vi "Delete.vi"(8 "error in":errorcluster, 11 "Driver path":path) -> (0 "error out":errorcluster)   [LabVIEW 2020, in "r307-python-labview-driver.lvlib"]
uses:
  r307-python-labview-driver.lvlib
  <vilib>/Utility/error.llb/whitespace.ctl
panel:
  out "standard error":string
  out "standard output":string
  in  "Enrolled ID":u32
  out "Deleted":bool
  out "command line":string="cmc /c python \"%s\" ENROLL"
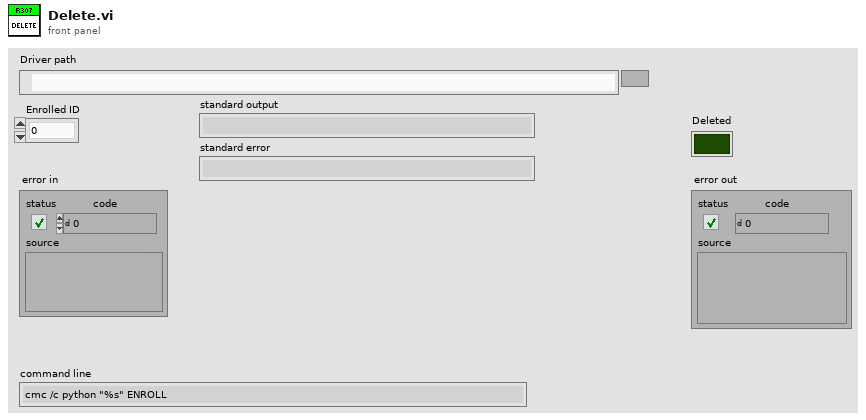
[diagram p1: front panel]
types:
  T1 = typedef "whitespace.ctl" = u16
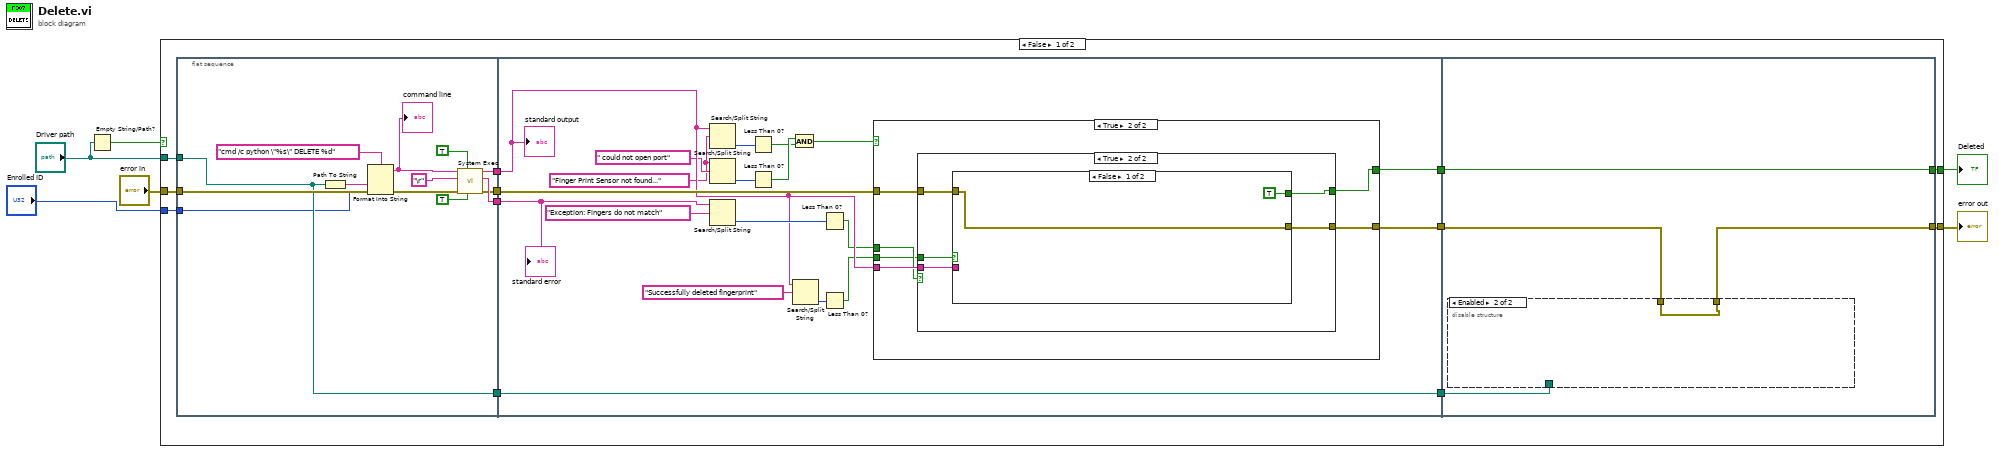
[diagram p0: block diagram]
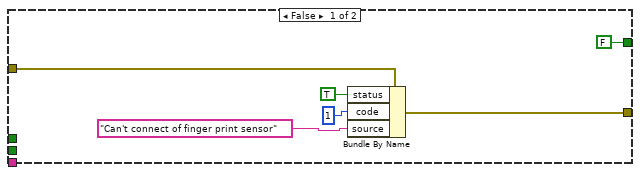
[diagram p2: hidden frame]
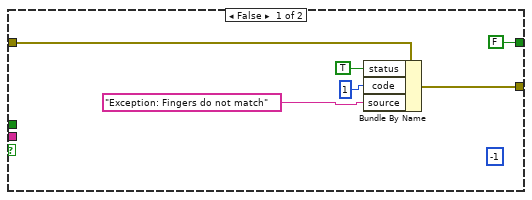
[diagram p3: hidden frame]
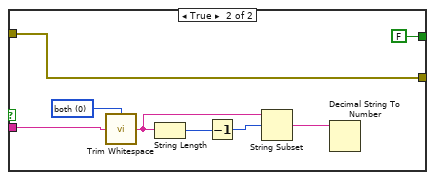
[diagram p4: hidden frame]
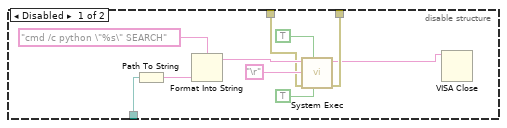
[diagram p5: hidden frame]
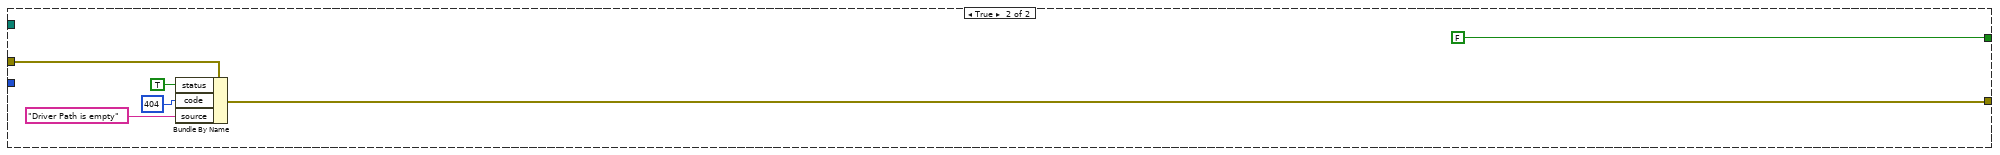
[diagram p6: hidden frame]
diagram:
  n1 = Empty String/Path?(string/path="Driver path") -> (empty?=w3:bool)
  n2 = case shown="False" w3 {
    tunnel: "Driver path" -> [w15 _]
    tunnel: "error in" -> [w14 w103]
    tunnel: [w13 w99] -> w5
    tunnel: [w12 FALSE ("Found")] -> w4
    tunnel: "Enrolled ID" -> [w7 _]
    frame False {
      n3 = flat-sequence {
        tunnel: w15 -> [w20]
        tunnel: w14 -> [w22]
        tunnel: [w25] -> w18
        tunnel: [w21] -> w17
        tunnel: [w24] -> w16
        tunnel: [w20] -> w8
        tunnel: w7 -> [w19]
        tunnel: w18 -> [w48]
        tunnel: w17 -> [w47]
        tunnel: w16 -> [w41]
        tunnel: [w43] -> w11
        tunnel: [w39] -> w10
        tunnel: [w32] -> w9
        tunnel: w8 -> [w32]
        tunnel: [w86] -> w12
        tunnel: [w83] -> w13
        tunnel: w11 -> [w84]
        tunnel: w10 -> [w86]
        tunnel: w9 -> [w85]
        frame #0 {
          n4 = Path To String(path=w20) -> (string=w27:string)
          n5 = Format Into String(format string="cmd /c python \"%s\" DELETE %d" ("command line"), w27, w19) -> (resulting string=w28:string)  [unwired: 2 in, 1 out]
          "command line" <- w28
          n6 = call <vilib>:"System Exec.vi"("run minimized? (F)"=TRUE, "wait until completion? (T)"=TRUE, "error in (no error)"=w22, "standard input"="\r", "command line"=w28) -> ("error out"=w21:errorcluster, "standard error"=w25:string, "standard output"=w24:string)  [unwired: 3 in, 1 out]
        }
        frame #1 {
          w33 = "Finger Print Sensor not found..." ("search string/char (-)")
          n7 = Search/Split String(string=w41, search string/char (-)=w33) -> (offset of match=w46:i32)  [unwired: 1 in, 2 out]
          n8 = Search/Split String(string=w33, search string/char (-)=" could not open port") -> (offset of match=w38:i32)  [unwired: 1 in, 2 out]
          n9 = Search/Split String(string=w48, search string/char (-)="Exception: Fingers do not match") -> (offset of match=w49:i32)  [unwired: 1 in, 2 out]
          n10 = Less Than 0?(x=w46) -> (x < 0?=w36:bool)
          n11 = Less Than 0?(x=w38) -> (x < 0?=w37:bool)
          n12 = And(x=w37, y=w36) -> (x .and. y?=w35:bool)
          n13 = Search/Split String(string=w41, search string/char (-)="Successfully deleted fingerprint" ("string")) -> (offset of match=w45:i32)  [unwired: 1 in, 2 out]
          n14 = Less Than 0?(x=w49) -> (x < 0?=w40:bool)
          n15 = Less Than 0?(x=w45) -> (x < 0?=w31:bool)
          n16 = case shown="True" w35 {
            tunnel: w47 -> [w52 w61]
            tunnel: w41 -> [_ w59]
            tunnel: [w51 w60] -> w43
            tunnel: w40 -> [_ w58]
            tunnel: w31 -> [_ w57]
            tunnel: [FALSE ("Found") w56] -> w39
            frame False {
              n17 = Bundle By Name(cluster=w52, "status"=TRUE, "code"=1, "source"="Can't connect of finger print sensor" ("search string/char (-)")) -> (w51:errorcluster)
            }
            frame True {
              n18 = case shown="True" w58 {
                tunnel: w61 -> [w67 w70]
                tunnel: [w64 w69] -> w60
                tunnel: w59 -> [_ w72]
                tunnel: w57 -> [_ w71]
                tunnel: [FALSE ("Found") w68] -> w56
                frame False {
                  (unwired) -1 ("Enrolled ID")
                  n19 = Bundle By Name(cluster=w67, "status"=TRUE, "code"=1, "source"="Exception: Fingers do not match" ("search string/char (-)")) -> (w64:errorcluster)
                }
                frame True {
                  n20 = case shown="False" w71 {
                    tunnel: w72 -> [_ w77]
                    tunnel: w70 -> [w74 w79]
                    tunnel: [w74 w79] -> w69
                    tunnel: [TRUE ("Found") FALSE ("Found")] -> w68
                    frame False {
                    }
                    frame True {
                      w78 = T1 0 items=["both", "start of string", "end of string"] ("location (both)")
                      n21 = call <vilib>:"Trim Whitespace.vi"("string"=w77, "location (both)"=w78) -> ("trimmed string"=w76:string)
                      n22 = String Length(string=w76) -> (length=w81:i32)
                      n23 = Decrement(x=w81) -> (x-1=w80:i32)
                      n24 = String Subset(string=w76, offset (0)=w80) -> (substring=w82:string)  [unwired: 1 in]
                      n25 = Decimal String To Number(string=w82) -> ()  [unwired: 2 in, 2 out]
                    }
                  }
                }
              }
            }
          }
          "standard output" <- w41
          "standard error" <- w48
        }
        frame #2 {
          n26 = disable-structure shown="Enabled" {
            disable-tunnel: w85 -> [w90 _]
            disable-tunnel: w84 -> [w89 w97]
            disable-tunnel: [w88 w97] -> w83
            frame Disabled {
              n27 = Path To String(path=w90) -> (string=w95:string)
              n28 = Format Into String(format string="cmd /c python \"%s\" SEARCH" ("command line"), w95) -> (resulting string=w96:string)  [unwired: 2 in, 1 out]
              n29 = call <vilib>:"System Exec.vi"("run minimized? (F)"=TRUE, "wait until completion? (T)"=TRUE, "error in (no error)"=w89, "standard input"="\r", "command line"=w96) -> ("error out"=w88:errorcluster, "standard output"=w87:string)  [unwired: 3 in, 2 out]
              n30 = VISA Close(VISA resource name=w87) -> ()  [unwired: 1 in, 1 out]
            }
            frame Enabled {
            }
          }
        }
      }
    }
    frame True {
      n31 = Bundle By Name(cluster=w103, "status"=TRUE, "code"=404, "source"="Driver Path is empty") -> (w99:errorcluster)
    }
  }
  "error out" <- w5
  "Deleted" <- w4
